vi "Serial Write and Read on Two Ports.vi"() -> ()   [LabVIEW 2013]
doc: "This example opens two VISA resources and configures one COM port to perform a write operation and the other COM port to perform a read operation. This VI will wait until the specified number of bytes is received at the port or until a termination character is read.\n\nThis example allows you perform diagnostic tests on your ports. You can use this example to perform a wrap-back test. Both serial ports must have the same basic configuration parameters. You can connect two of the ports using a null modem cable, which effectively connects one port's RX lines to the other port's TX lines. If you use a straight-through cable, one port's RX lines will be connected to the other port's RX lines, and you cannot communicate between the two ports."
uses:
  <vilib>/Instr/_visa.llb/VISA Configure Serial Port (Instr).vi
panel:
  in  "WAIT(ms)":u32
  in  "?":bool
  in  "Write String":string="*IDN?"
  out "Read String":string
  in  "VISA Resource (write)":refnum<visa-resource-name>="COM1"
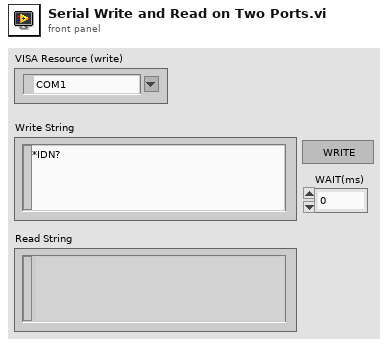
[diagram p1: front panel]
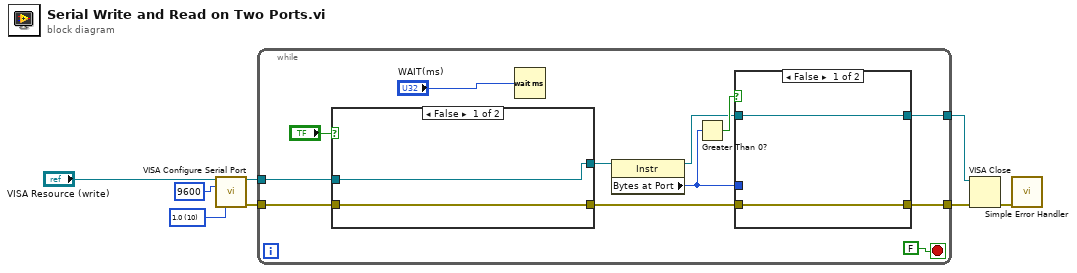
[diagram p0: block diagram]
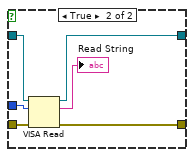
[diagram p2: hidden frame]
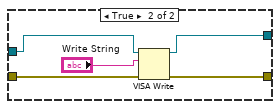
[diagram p3: hidden frame]
diagram:
  w1 = u16 10 items=["1.0"=10, "1.5"=15, "2.0"=20] ("stop bits (10: 1 bit)")
  n1 = call-poly "VISA Configure Serial Port"("VISA resource name"="VISA Resource (write)", "baud rate (9600)"=u32 9600, "stop bits (10: 1 bit)"=w1) -> ("VISA resource name out"=w3:refnum<visa-resource-name>, "error out"=w2:errorcluster)  [unwired: 6 in, 5 out]
  n2 = while {
    tunnel: [w20] -> w7
    tunnel: w2 -> [w18]
    tunnel: w3 -> [w16]
    tunnel: [w12] -> w5
    stop <- FALSE stop-if-true
    n3 = case shown="False" "?" {
      tunnel: [w29 w35] -> w19
      tunnel: w16 -> [w30 w33]
      tunnel: w18 -> [w29 w32]
      tunnel: [w30 w31] -> w14
      frame False {
      }
      frame True {
        n4 = VISA Write(VISA resource name=w33, write buffer="Write String", error in (no error)=w32) -> (VISA resource name out=w31:refnum<visa-resource-name>, error out=w35:errorcluster)  [unwired: 1 out]
      }
    }
    n5 = Wait (ms)(milliseconds to wait="WAIT(ms)") -> ()  [unwired: 1 out]
    n6 = property class="Instr"(reference=w14) -> (reference out=w13:refnum<visa-resource-name>, "Bytes at Port"=w10:u32)  [unwired: 1 in, 1 out]
    n7 = Greater Than 0?(x=w10) -> (x > 0?=w15:bool)
    n8 = case shown="False" w15 {
      tunnel: [w22 w28] -> w20
      tunnel: w19 -> [w21 w27]
      tunnel: w13 -> [w22 w26]
      tunnel: [w21 w24] -> w12
      tunnel: w10 -> [_ w23]
      frame False {
      }
      frame True {
        n9 = VISA Read(VISA resource name=w26, byte count=w23, error in (no error)=w27) -> (VISA resource name out=w28:refnum<visa-resource-name>, read buffer=→"Read String":string, error out=w24:errorcluster)  [unwired: 1 out]
      }
    }
  }
  n10 = VISA Close(VISA resource name=w7, error in (no error)=w5) -> (error out=w6:errorcluster)
  n11 = call <vilib>:"Simple Error Handler.vi"("error in (no error)"=w6) -> ()  [unwired: 1 in, 8 out]
